vi "ExposeParseObjectMapNamePath.vi"(11 "MatlabDataBundle":T1) -> (3 "Name parts array":string[](array[string]))   [LabVIEW 2017]
uses:
  ExposeObjectMapNamepathData.ctl
  ExposeMapperDataTypeEnum.ctl
  ExposeObjectMapContainerTypeEnum.ctl
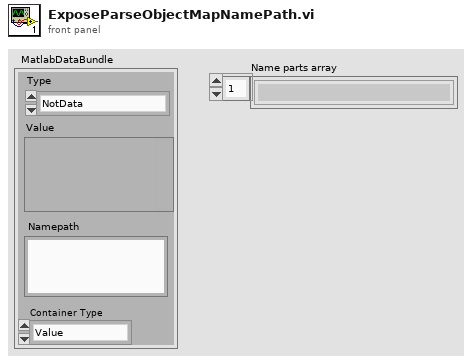
[diagram p1: front panel]
types:
  T1 = typedef "ExposeObjectMapNamepathData.ctl" = cluster{"Type":T2, "Value":variant, "Namepath":string, "Container Type":T3}
  T2 = typedef "ExposeMapperDataTypeEnum.ctl" = enum16{"NotData", "Real", "Complex", "String", "Boolean", "Container"}
  T3 = typedef "ExposeObjectMapContainerTypeEnum.ctl" = enum16{"Value", "Array", "Waveform", "NetContainer"}
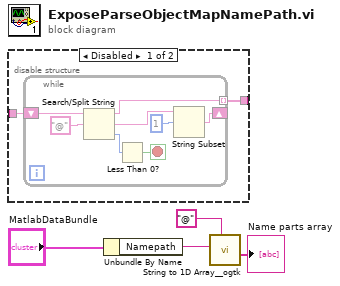
[diagram p0: block diagram]
diagram:
  n1 = disable-structure shown="Disabled" {
    disable-tunnel: [w6 _] -> _
    disable-tunnel: _ -> [w5 _]
    frame Disabled {
      n2 = while {
        tunnel: [w13] -> w6 mode=indexing
        shift-right: [w7] -> _
        shift-left: w5 -> [w10]
        stop <- w11 stop-if-true
        n3 = Search/Split String(string=w10, search string/char (-)="@") -> (substring before match=w13:string, match + rest of string=w8:string, offset of match=w12:i32)  [unwired: 1 in]
        n4 = Less Than 0?(x=w12) -> (x < 0?=w11:bool)
        n5 = String Subset(string=w8, offset (0)=1) -> (substring=w7:string)  [unwired: 1 in]
      }
    }
    frame Enabled {
    }
  }
  n6 = Unbundle By Name("MatlabDataBundle") -> ("Namepath"=w3:string)
  n7 = call <userlib>:"String to 1D Array__ogtk.vi"("delimiter (Tab)"="@" ("search string/char (-)"), "string"=w3) -> ("Array of Strings"=→"Name parts array":string[])  [unwired: 9 in]
